vi "New SinglePlotPanel Type.vi"(8 "error in (no error)":errorcluster, 10 "Init options":T1={"UI visible?"=FALSE, "Update rate (ms)"=250, "Sidebar.Visible"=TRUE, "time to plot (init)"=600.0, "time to plot (max)"=inf, "config file start path"=path "", "Title.Visible"=TRUE, "Title"="Title", "TimeZone"=enum."Local"} {"time to plot (init)" format="%<%H:%M:%S>t"}, 11 "BluePlotHandle":refnum<class "RocketPlotHandle.lvclass">) -> (0 "error out":errorcluster, 3 "SinglePlotPanel out":refnum<class "RocketPlotPanel.lvclass">)   [LabVIEW 2021, in "RocketPlot.lvlib" / "RocketPlotPanel.lvclass"]
uses:
  RocketPlotPanel.lvclass
  RocketPlotHandle/SubVIs/Init Options.ctl
  TypeDefs/TimeZone.ctl
  RocketPlotHandle/RocketPlotHandle.lvclass
  RocketPlotPanel.lvclass/RocketPlotPanel.ctl
  TypeDefs/panel mode.ctl
  RocketPlot.lvlib
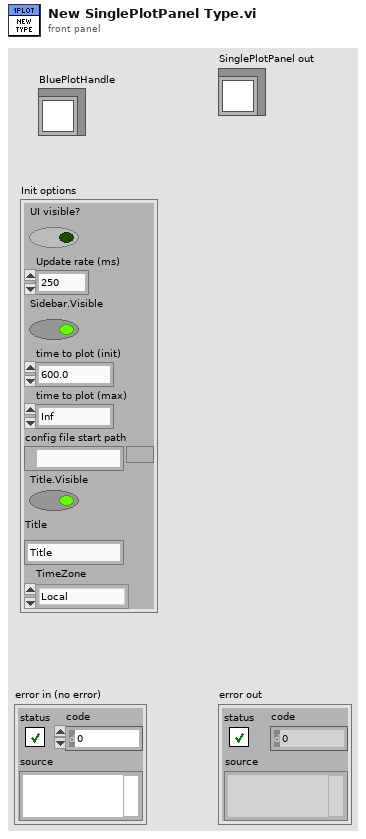
[diagram p1: front panel]
types:
  T1 = typedef "RocketPlotHandle.lvclass/Init Options.ctl" = cluster{"UI visible?":bool, "Update rate (ms)":u32, "Sidebar.Visible":bool, "time to plot (init)":dbl, "time to plot (max)":dbl, "config file start path":path, "Title.Visible":bool, "Title":string, "TimeZone":T2}
  T2 = typedef "RocketPlot.lvlib/TimeZone.ctl" = enum16{"UTC", "Local"}
  T3 = typedef "RocketPlot.lvlib/panel mode.ctl" = enum16{"1PLOT", "MPLOT"}
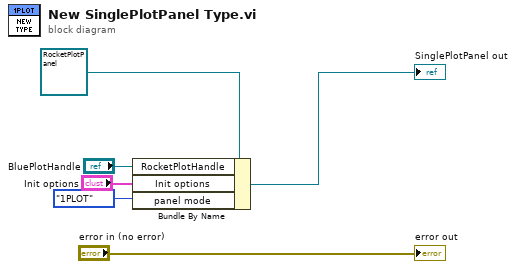
[diagram p0: block diagram]
diagram:
  n1 = Bundle By Name(cluster=refnum<class "RocketPlotPanel.lvclass"> refnum ("SinglePlotPanel out"), "RocketPlotHandle"="BluePlotHandle", "Init options"="Init options", "panel mode"=panel_mode."1PLOT") -> (→"SinglePlotPanel out":refnum<class "RocketPlotPanel.lvclass">)
  "error out" <- "error in (no error)"
